vi "AB_API Add Destination.vi"(8 "error in (no error)":errorcluster, 9 "Destination type (directory)":T1, 10 "Destination label":string, 11 "Build in":refnum<class "AB_Build.lvclass">) -> (0 "error out":errorcluster, 3 "Build out":refnum<class "AB_Build.lvclass">)   [LabVIEW 2020]
uses:
  <vilib>/AppBuilder/AB_Classes/Build/AB_Build.lvclass
  <vilib>/AppBuilder/AB_API/common/AB_API Destination Type.ctl
  <vilib>/AppBuilder/AB_Destination_Type.ctl
  <vilib>/AppBuilder/AB_Classes/Destination/AB_Destination.lvclass
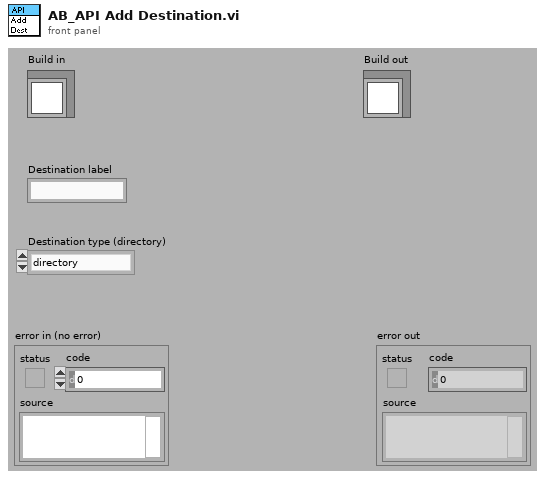
[diagram p1: front panel]
types:
  T1 = typedef "AB_API Destination Type.ctl" = enum16{"directory", "directory (preserve hierarchy)", "LLB"}
  T2 = typedef "AB_Destination_Type.ctl" = enum32{"No Selection", "Directory", "LLB"}
  T3 = typedef "AB_Build.ctl" = cluster{"buildSpecName":string, "buildSpecDescription":string, "destinations":refnum<class "AB_Destination.lvclass">[], "exclusionOption":T4, "defaultLanguage":string, "supportedLanguages":string[], "excludedDirectories":path[], "buildContext":refnum<vi>, "buildObject":T5, "preview":bool, "programatic":bool, "progressBarEvents":T6, "userLog_Path":path, "preActionID":string, "preAction_Path":path, "postActionID":string, "postAction_Path":path, "eng_checkForBrokenVIs?":bool, "eng_verboseLinkerErrors?":bool, "localDest_Path":path, "targetDest_Path":path, "removeVIObject":u16, "cache":refnum<class "PreviewCache.lvclass">, "use cache":bool, "previewCache_ID":string, "buildCache_ID":string, "eng_TempLocalDest_Path":path, "eng_collectDependencies?":bool, "versionInfo":cluster{"buildVersion":cluster{"major":u16, "minor":u16, "patch":u16, "build":u16}, "autoIncrement":bool}, "eng_enableVIChecksums":bool}
  T4 = typedef "AB_Exclusion_Option.ctl" = cluster{"typedefs":bool, "polymorphicVIs":bool, "unusedLibraryItems":bool, "modifyLibraryFile":bool, "edit-timeDependencies":bool, "inlineVIs":bool, "dependent PPLs":bool, "dependent DLLs":bool}
  T5 = typedef "ItemRef.ctl" = u64
  T6 = typedef "provcom_ProgressBar_Events.ctl" = cluster{"newJob":refnum<user-event>, "newItem":refnum<user-event>, "errorMsg":T7, "cancel":refnum<user-event>}
  T7 = typedef "mxLvBuildError.ctl" = refnum<user-event>
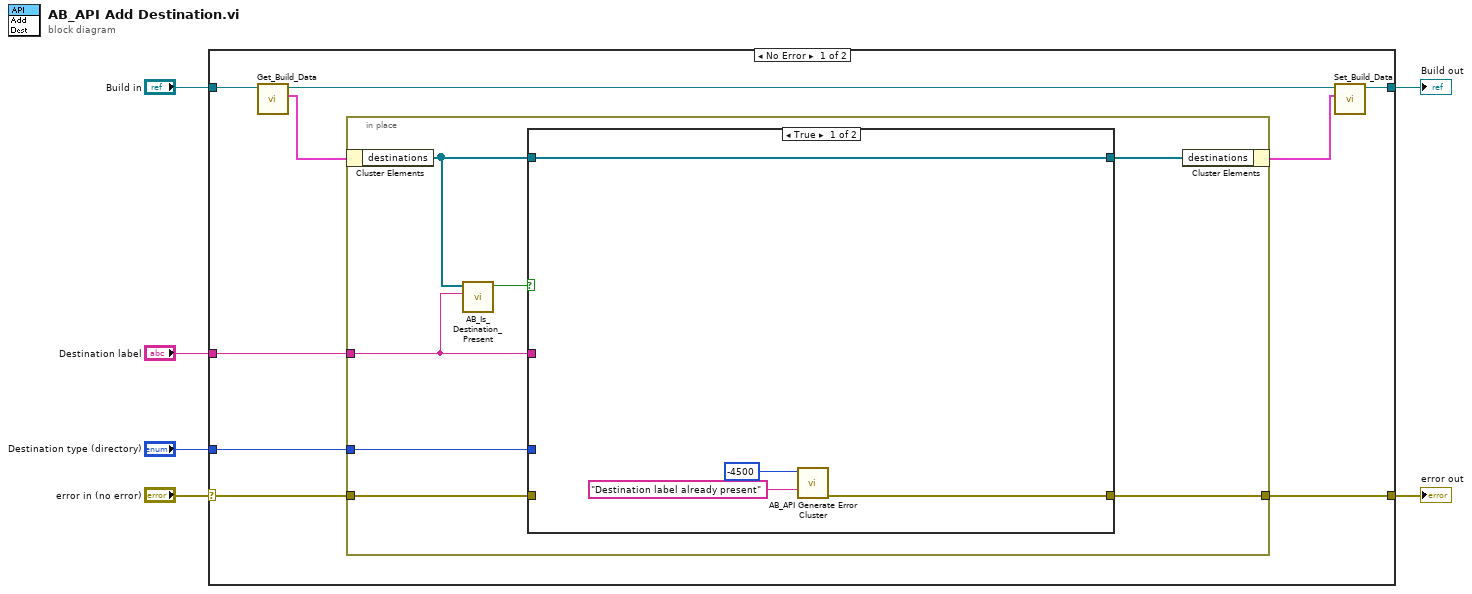
[diagram p0: block diagram]
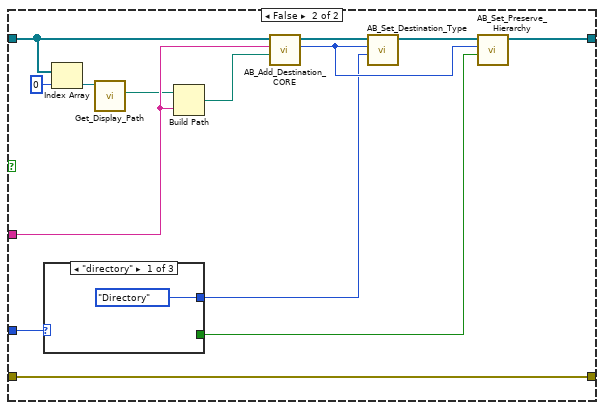
[diagram p2: hidden frame]
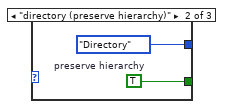
[diagram p3: hidden frame]
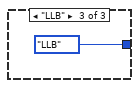
[diagram p4: hidden frame]
diagram:
  n1 = case shown="No Error" "error in (no error)" {
    selector: "error in (no error)" -> [w10 w46]
    tunnel: [w9 w46] -> w5
    tunnel: "Build in" -> [w12 w45]
    tunnel: [w11 w45] -> w3
    tunnel: "Destination label" -> [w8 _]
    tunnel: "Destination type (directory)" -> [w7 _]
    frame No Error {
      n2 = call <vilib>:"Get_Build_Data.vi"("Class in"=w12) -> ("data"=w14:T3, "Class out"=w15:refnum<class "AB_Build.lvclass">)  [unwired: 1 in, 8 out]
      n3 = in-place {
        in-place-border: w8 -> [w16]
        in-place-border: w7 -> [w21]
        in-place-border: [w20] -> w9
        in-place-border: w10 -> [w19]
        n4 = in-place-cluster #1(w14) -> ("destinations"=w18:refnum<class "AB_Destination.lvclass">[])
        n5 = call <vilib>:"AB_Is_Destination_Present.vi"("destination label"=w16, "destinations"=w18) -> ("destination present?"=w17:bool)  [unwired: 1 in, 8 out]
        n6 = case shown="True" w17 {
          tunnel: [w26 w39] -> w22
          tunnel: w18 -> [w26 w33]
          tunnel: w16 -> [_ w38]
          tunnel: w21 -> [_ w29]
          tunnel: [w24 w40] -> w20
          tunnel: w19 -> [_ w40]
          frame True {
            n7 = call <vilib>:"AB_API Generate Error Cluster.vi"("Additional Message"="Destination label already present", "Code"=-4500) -> ("error out"=w24:errorcluster)  [unwired: 2 in, 7 out]
          }
          frame False {
            n8 = case shown="\"directory\"" w29 {
              tunnel: [AB_Destination_Type."Directory" ("destination type") AB_Destination_Type."Directory" ("destination type") AB_Destination_Type."LLB" ("destination type")] -> w28
              tunnel: [_ w42 _] -> w27
              frame "directory" {
              }
              frame "directory (preserve hierarchy)" {
                w42 = TRUE  # preserve hierarchy
              }
              frame "LLB" {
              }
            }
            n9 = Index Array(array=w33, index=0) -> (element=w36:refnum<class "AB_Destination.lvclass">)
            n10 = call-dynamic "Get_Display_Path.vi"("AB_Destination in"=w36) -> ("displayPath"=w34:path)  [unwired: 1 in, 9 out]
            n11 = Build Path(base path=w34, name or relative path=w38) -> (appended path=w37:path)
            n12 = call <vilib>:"AB_Add_Destination_CORE.vi"("destination path"=w37, "destination label"=w38, "destinations in"=w33) -> ("destination index"=w32:i32, "destinations out"=w31:refnum<class "AB_Destination.lvclass">[])  [unwired: 4 in, 3 out]
            n13 = call <vilib>:"AB_Set_Destination_Type.vi"("destination type"=w28, "destination index"=w32, "destinations in"=w31) -> ("destinations out"=w30:refnum<class "AB_Destination.lvclass">[])  [unwired: 1 in, 7 out]
            n14 = call <vilib>:"AB_Set_Preserve_Hierarchy.vi"("preserve hierarchy"=w27, "destination index"=w32, "destinations in"=w30) -> ("destinations out"=w39:refnum<class "AB_Destination.lvclass">[])  [unwired: 1 in, 7 out]
          }
        }
        n15 = in-place-cluster #1("destinations"=w22) -> (w13:T3)
      }
      n16 = call <vilib>:"Set_Build_Data.vi"("data"=w13, "Class in"=w15) -> ("Class out"=w11:refnum<class "AB_Build.lvclass">)  [unwired: 1 in, 8 out]
    }
    frame Error {
    }
  }
  "error out" <- w5
  "Build out" <- w3
